vi "Strings und Zeitstempel verknuepfen.vi"(8 "String 2 hinzufügen":string, 9 "String 1 hinzufügen":string, 11 "Eingagns String":string) -> (2 "Verknüpfter String":string)   [LabVIEW 2020, in "FT-IR.lvlib"]
uses:
  FT-IR.lvlib
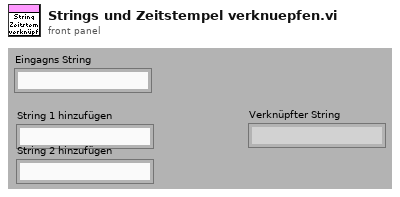
[diagram p1: front panel]
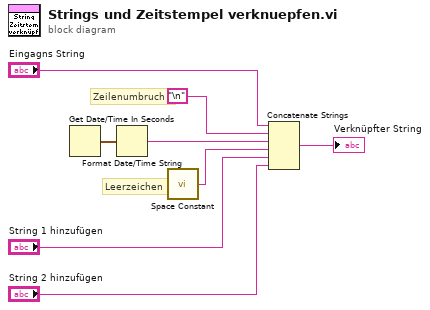
[diagram p0: block diagram]
diagram:
  # "Leerzeichen"
  # "Zeilenumbruch"
  n1 = Get Date/Time In Seconds() -> (seconds since 1Jan1904=w7:timestamp)
  n2 = Format Date/Time String(seconds (now)=w7) -> (date/time string=w6:string)  [unwired: 2 in]
  n3 = call <vilib>:"Space Constant.vi"() -> ("String"=w5:string)
  n4 = Concatenate Strings("Eingagns String", "\n", w6, w5, "String 1 hinzufügen", "String 2 hinzufügen") -> (→"Verknüpfter String":string)
